vi "Test - 7.vi"() -> ()   [LabVIEW 2013]
uses:
  Item/Ctls/Item Reference.ctl
  Channel/Ctls/ChannelSetting.ctl
  Channel/Ctls/IOType.ctl
  Channel/Ctls/Dimensions.ctl
  <vilib>/Utility/sysdir.llb/System Directory Type.ctl
  Section/Section.lvclass
  Channel/Channel.lvclass
  Item/Item.lvclass
panel:
  in  "树形":string(tree)
  out "Property Names":string[](array[string])
  out "Values":variant[](array[variant])
  out "Children Item Names":string[](array[string])
  out "Newly Created?":bool
  in  "刷新按钮":bool
  in  "Name":string
  out "found":bool
  out "PathName":string
  out "Address":string
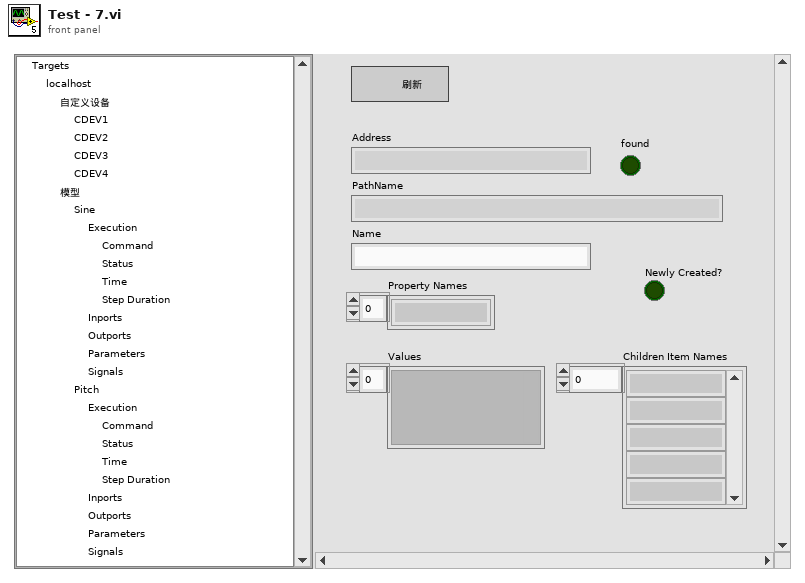
[diagram p1: front panel]
types:
  T1 = typedef "Hierarchy Framework.lvlib/Item.lvclass/Item Reference.ctl" = u64
  T2 = cluster{"Left Cell String":string, "Child Text":string[], "Child Tag":string, "Item Indent":i32, "Child Only?":bool, "Glyph Index":i32}[]
  T3 = cluster{"SectionName":string, "TypeGUID":string}[]
  T4 = typedef "Hierarchy Framework.lvlib/Channel.lvclass/ChannelSetting.ctl" = cluster{"IOType":T5, "DefaultValue":dbl[][], "Dimensions":T6, "Units":string, "Description":string, "Faultable":bool}
  T5 = typedef "Hierarchy Framework.lvlib/Channel.lvclass/IOType.ctl" = enum16{"Input", "Output"}
  T6 = typedef "Hierarchy Framework.lvlib/Channel.lvclass/Dimensions.ctl" = cluster{"Row":i32, "Column":i32}
  T7 = cluster{"Channel Name":string, "Channel Setting":T4}[]
  T8 = typedef "System Directory Type.ctl" = i32
  T9 = typedef "Hierarchy Framework.lvlib/Item.lvclass/Item Info.ctl" = cluster{"Name":string, "TagGUID":string, "TypeGUID":string, "Enable":bool}
  T10 = typedef "LVPoint32TypeDef.ctl" = cluster{"Horizontal":i32, "Vertical":i32}
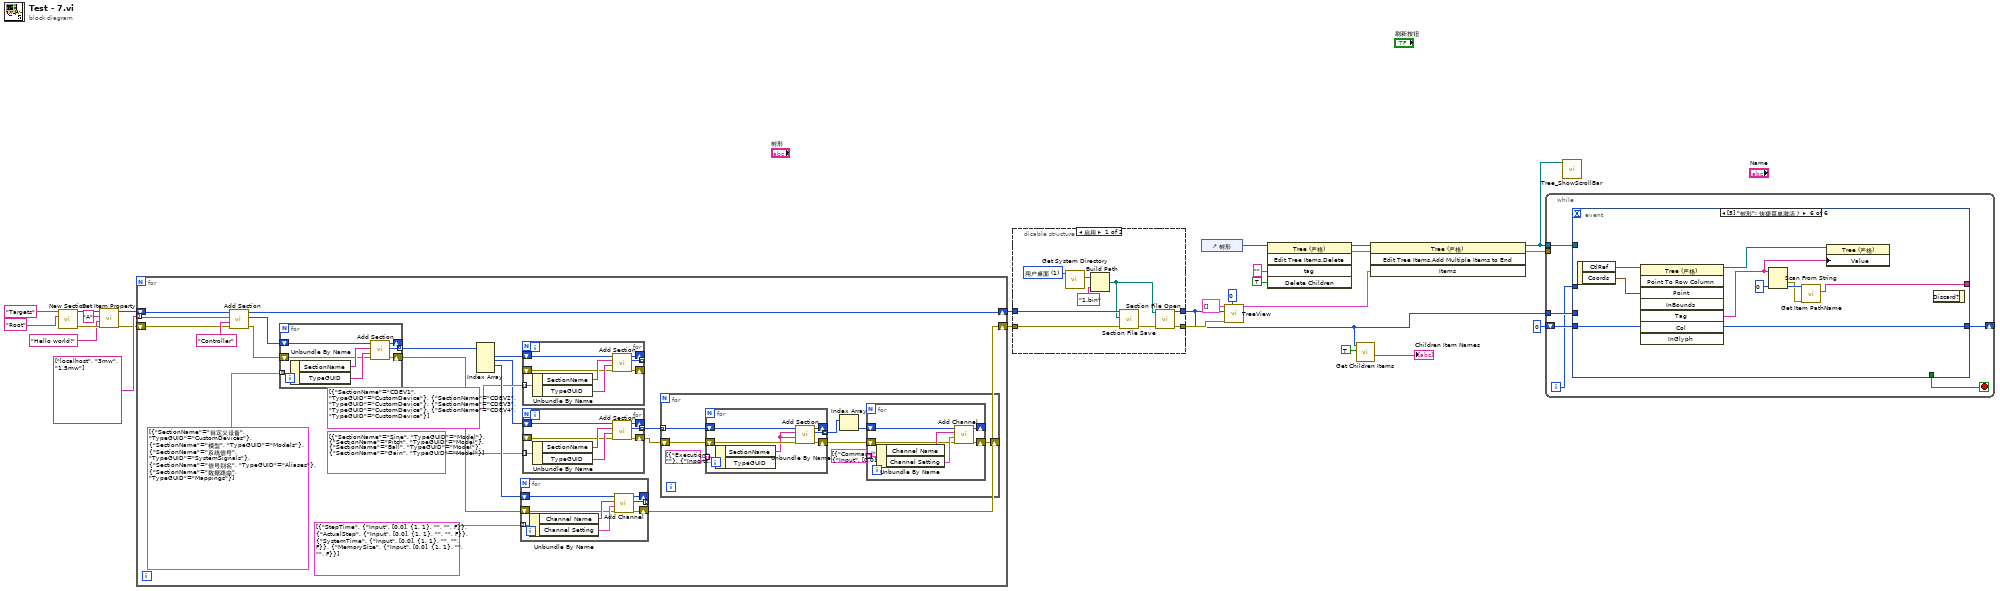
[diagram p0: block diagram]
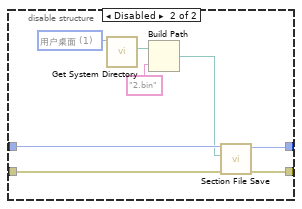
[diagram p2: hidden frame]
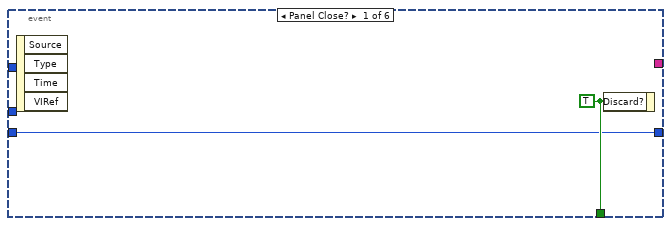
[diagram p3: hidden frame]
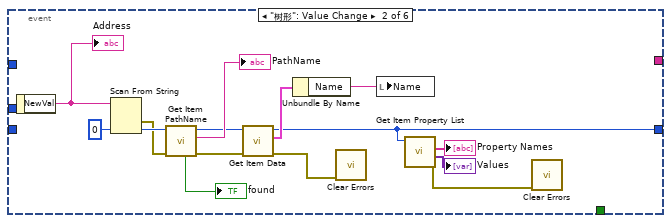
[diagram p4: hidden frame]
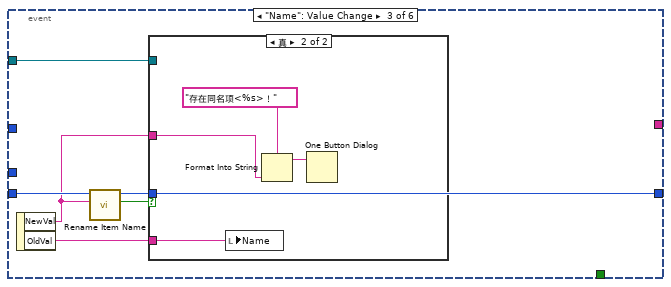
[diagram p5: hidden frame]
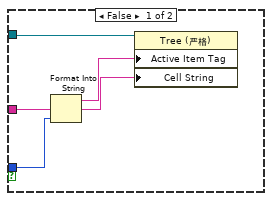
[diagram p6: hidden frame]
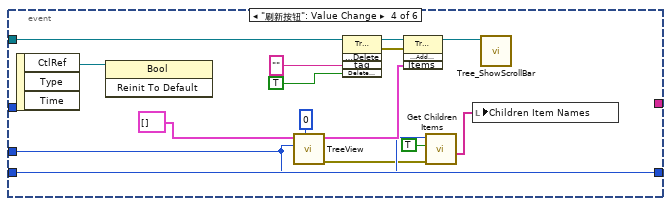
[diagram p7: hidden frame]
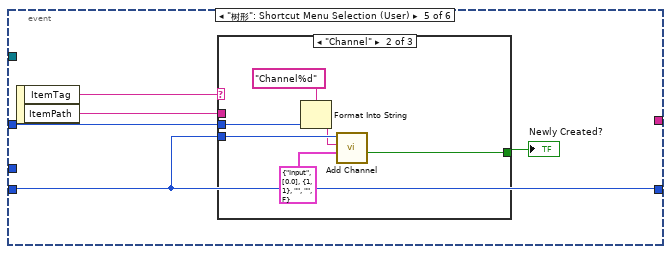
[diagram p8: hidden frame]
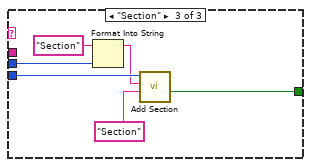
[diagram p10: hidden frame]
diagram:
  n1 = call "New Section.vi"("TypeGUID"="Root" ("Name"), "Name"="Targets") -> ("error out"=w6:errorcluster, "Section Reference in"=w8:u64)  [unwired: 8 in]
  n2 = call "Set Item Property.vi"("error in (no error)"=w6, "Value"="Hello world!" ("Property Name"), "Property Name"="A", "Item Reference in"=w8) -> ("error out"=w5:errorcluster, "Item Reference out"=w7:T1)  [unwired: 5 in, 1 out]
  n3 = for {
    shift-right: [w37] -> w2
    shift-left: w7 -> [w35]
    shift-right: [w36] -> w10
    shift-left: w5 -> [w34]
    tunnel: string[] ["localhost", "3mw", "1.5mw"] -> [w33] mode=indexing
    n4 = call "Add Section.vi"("error in (no error)"=w34, "TypeGUID"="Controller" ("SectionName"), "SectionName"=w33, "Section Reference in"=w35) -> ("error out"=w39:errorcluster, "Section Reference"=w44:u64, "Section Reference out"=w37:u64)  [unwired: 4 in, 1 out]
    n5 = for {
      shift-right: [w98] -> _
      shift-left: w44 -> [w99]
      tunnel: T3 [{"SectionName"="自定义设备", "TypeGUID"="CustomDevices"}, {"SectionName"="模型", "TypeGUID"="Models"}, {"SectionName"="系统信号", "TypeGUID"="SystemSignals"}, {"SectionName"="信号别名", "TypeGUID"="Aliases"}, {"SectionName"="数据路由", "TypeGUID"="Mappings"}] -> [w97] mode=indexing
      tunnel: [w94] -> w42 mode=indexing
      shift-right: [w92] -> w38
      shift-left: w39 -> [w93]
      n6 = Unbundle By Name(w97) -> ("SectionName"=w96:string, "TypeGUID"=w95:string)
      n7 = call "Add Section.vi"("error in (no error)"=w93, "TypeGUID"=w95, "SectionName"=w96, "Section Reference in"=w99) -> ("error out"=w92:errorcluster, "Section Reference"=w94:u64, "Section Reference out"=w98:u64)  [unwired: 4 in, 1 out]
    }
    n8 = Index Array(array=w42) -> (element #1=w32:u64, element #2=w30:u64, element #3=w40:u64)  [unwired: 4 in, 1 out]
    n9 = for {
      shift-right: [w90] -> _
      shift-left: w40 -> [w91]
      tunnel: T7 [{"Channel Name"="StepTime", "Channel Setting"={"IOType"=enum."Input", "DefaultValue"=[[0.0]], "Dimensions"={"Row"=1, "Column"=1}, "Units"="", "Description"="", "Faultable"=FALSE}}, {"Channel Name"="ActualStep", "Channel Setting"={"IOType"=enum."Input", "DefaultValue"=[[0.0]], "Dimensions"={"Row"=1, "Column"=1}, "Units"="", "Description"="", "Faultable"=FALSE}}, {"Channel Name"="SystemTime", "Channel Setting"={"IOType"=enum."Input", "DefaultValue"=[[0.0]], "Dimensions"={"Row"=1, "Column"=1}, "Units"="", "Description"="", "Faultable"=FALSE}}, {"Channel Name"="MemorySize", "Channel Setting"={"IOType"=enum."Input", "DefaultValue"=[[0.0]], "Dimensions"={"Row"=1, "Column"=1}, "Units"="", "Description"="", "Faultable"=FALSE}}] -> [w89] mode=indexing
      tunnel: [w86] -> _ mode=indexing
      shift-right: [w84] -> w36
      shift-left: w38 -> [w85]
      n10 = Unbundle By Name(w89) -> ("Channel Name"=w88:string, "Channel Setting"=w87:T4)
      n11 = call "Add Channel.vi"("error in (no error)"=w85, "Channel Setting"=w87, "Channel Name"=w88, "Section Reference in"=w91) -> ("error out"=w84:errorcluster, "Channel Reference"=w86:u64, "Section Reference out"=w90:u64)  [unwired: 4 in, 1 out]
    }
    n12 = for {
      shift-right: [w82] -> _
      shift-left: w32 -> [w83]
      tunnel: T3 [{"SectionName"="CDEV1", "TypeGUID"="CustomDevice"}, {"SectionName"="CDEV2", "TypeGUID"="CustomDevice"}, {"SectionName"="CDEV3", "TypeGUID"="CustomDevice"}, {"SectionName"="CDEV4", "TypeGUID"="CustomDevice"}] -> [w81] mode=indexing
      tunnel: [w78] -> _ mode=indexing
      shift-right: [w76] -> _
      shift-left: _ -> [w77]
      n13 = Unbundle By Name(w81) -> ("SectionName"=w80:string, "TypeGUID"=w79:string)
      n14 = call "Add Section.vi"("error in (no error)"=w77, "TypeGUID"=w79, "SectionName"=w80, "Section Reference in"=w83) -> ("error out"=w76:errorcluster, "Section Reference"=w78:u64, "Section Reference out"=w82:u64)  [unwired: 4 in, 1 out]
    }
    n15 = for {
      shift-right: [w74] -> _
      shift-left: w30 -> [w75]
      tunnel: T3 [{"SectionName"="Sine", "TypeGUID"="Model"}, {"SectionName"="Pitch", "TypeGUID"="Model"}, {"SectionName"="Ball", "TypeGUID"="Model"}, {"SectionName"="Gain", "TypeGUID"="Model"}] -> [w73] mode=indexing
      tunnel: [w70] -> w28 mode=indexing
      shift-right: [w68] -> w27
      shift-left: _ -> [w69]
      n16 = Unbundle By Name(w73) -> ("SectionName"=w72:string, "TypeGUID"=w71:string)
      n17 = call "Add Section.vi"("error in (no error)"=w69, "TypeGUID"=w71, "SectionName"=w72, "Section Reference in"=w75) -> ("error out"=w68:errorcluster, "Section Reference"=w70:u64, "Section Reference out"=w74:u64)  [unwired: 4 in, 1 out]
    }
    n18 = for {
      tunnel: w28 -> [w53] mode=indexing
      shift-right: [w46] -> _
      shift-left: w27 -> [w52]
      n19 = for {
        shift-right: [w66] -> _
        shift-left: w53 -> [w67]
        tunnel: T3 [{"SectionName"="Execution", "TypeGUID"=""}, {"SectionName"="Inports", "TypeGUID"=""}, {"SectionName"="Outports", "TypeGUID"=""}, {"SectionName"="Parameters", "TypeGUID"=""}, {"SectionName"="Signals", "TypeGUID"=""}] -> [w65] mode=indexing
        tunnel: [w64] -> w50 mode=indexing
        shift-right: [w62] -> w47
        shift-left: w52 -> [w63]
        n20 = Unbundle By Name(w65) -> ("SectionName"=w61:string)  [unwired: 1 out]
        n21 = call "Add Section.vi"("error in (no error)"=w63, "TypeGUID"=w61, "SectionName"=w61, "Section Reference in"=w67) -> ("error out"=w62:errorcluster, "Section Reference"=w64:u64, "Section Reference out"=w66:u64)  [unwired: 4 in, 1 out]
      }
      n22 = Index Array(array=w50) -> (element=w49:u64)  [unwired: 1 in]
      n23 = for {
        shift-right: [w59] -> _
        shift-left: w49 -> [w60]
        tunnel: T7 [{"Channel Name"="Command", "Channel Setting"={"IOType"=enum."Input", "DefaultValue"=[[0.0]], "Dimensions"={"Row"=1, "Column"=1}, "Units"="", "Description"="", "Faultable"=FALSE}}, {"Channel Name"="Status", "Channel Setting"={"IOType"=enum."Input", "DefaultValue"=[[0.0]], "Dimensions"={"Row"=1, "Column"=1}, "Units"="", "Description"="", "Faultable"=FALSE}}, {"Channel Name"="Time", "Channel Setting"={"IOType"=enum."Input", "DefaultValue"=[[0.0]], "Dimensions"={"Row"=1, "Column"=1}, "Units"="", "Description"="", "Faultable"=FALSE}}, {"Channel Name"="Step Duration", "Channel Setting"={"IOType"=enum."Input", "DefaultValue"=[[0.0]], "Dimensions"={"Row"=1, "Column"=1}, "Units"="", "Description"="", "Faultable"=FALSE}}] -> [w58] mode=indexing
        shift-right: [w54] -> w46
        shift-left: w47 -> [w55]
        n24 = Unbundle By Name(w58) -> ("Channel Name"=w57:string, "Channel Setting"=w56:T4)
        n25 = call "Add Channel.vi"("error in (no error)"=w55, "Channel Setting"=w56, "Channel Name"=w57, "Section Reference in"=w60) -> ("error out"=w54:errorcluster, "Section Reference out"=w59:u64)  [unwired: 4 in, 2 out]
      }
    }
  }
  n26 = disable-structure shown="启用" {
    disable-tunnel: [w108 w112] -> w1
    disable-tunnel: w2 -> [w104 w113]
    disable-tunnel: w10 -> [w103 w111]
    disable-tunnel: [w100 w110] -> w9
    frame Enabled {
      w105 = T8 1 items=["用户目录"=0, "用户桌面"=1, "用户文档"=2, "用户应用程序数据"=3, "用户设置"=4, "用户临时目录"=5, "公共文档"=6, "公共应用程序数据"=7, "公共设置"=8, "公共缓存"=13, "系统核心库"=9, "系统安装库"=10, "应用程序文件"=11, "启动盘根目录"=12] ("system directory type")
      n27 = call <vilib>:"Get System Directory.vi"("system directory type"=w105) -> ("system directory"=w106:path)  [unwired: 10 in]
      n28 = Build Path(base path=w106, name or relative path="1.bin" ("名称或相对路径")) -> (appended path=w101:path)
      n29 = call "Section File Save.vi"("error in (no error)"=w103, "Section File Path"=w101, "Section Reference in"=w104) -> ("error out"=w102:errorcluster)  [unwired: 7 in, 1 out]
      n30 = call "Section File Open.vi"("error in (no error)"=w102, "Section File Path"=w101) -> ("error out"=w100:errorcluster, "Section Reference out"=w108:u64)  [unwired: 8 in]
    }
    frame Disabled {
      w114 = T8 1 items=["用户目录"=0, "用户桌面"=1, "用户文档"=2, "用户应用程序数据"=3, "用户设置"=4, "用户临时目录"=5, "公共文档"=6, "公共应用程序数据"=7, "公共设置"=8, "公共缓存"=13, "系统核心库"=9, "系统安装库"=10, "应用程序文件"=11, "启动盘根目录"=12] ("system directory type")
      n31 = call <vilib>:"Get System Directory.vi"("system directory type"=w114) -> ("system directory"=w115:path)  [unwired: 10 in]
      n32 = Build Path(base path=w115, name or relative path="2.bin" ("名称或相对路径")) -> (appended path=w109:path)
      n33 = call "Section File Save.vi"("error in (no error)"=w111, "Section File Path"=w109, "Section Reference in"=w113) -> ("error out"=w110:errorcluster, "Section Reference out"=w112:u64)  [unwired: 7 in]
    }
  }
  n34 = control-ref of="树形"() -> (w26:refnum<vi>)
  n35 = call "TreeView.vi"("Item Indent"=0, "error in (no error)"=w9, "Item Reference in"=w1, "Items in"=T2 []) -> ("Items out"=w19:T2)  [unwired: 6 in, 1 out]
  n36 = invoke class="Tree (严格)" method="Edit Tree Items.Delete"(reference=w26, "tag"="" ("标识符"), "Delete Children"=TRUE ("删除子项？")) -> (reference out=w20:refnum<vi>, error out=w21:errorcluster)  [unwired: 2 in, 3 out]
  n37 = call "Get Children Items.vi"("Whole Hierarchy?(F)"=TRUE ("Whole Indent?(F)"), "Section Reference in"=w1) -> ("Children Item Names"=→"Children Item Names":string[])  [unwired: 5 in, 4 out]
  n38 = invoke class="Tree (严格)" method="Edit Tree Items.Add Multiple Items to End"(reference=w20, error in=w21, "Items"=w19) -> (reference out=w13:refnum<vi>, error out=w17:errorcluster)  [unwired: 1 in, 2 out]
  n39 = while {
    tunnel: w17 -> [_]
    shift-right: [w121] -> _
    shift-left: T1 0 ("Item Reference out") -> [w120]
    tunnel: w13 -> [w119]
    tunnel: w1 -> [w118]
    i -> [w117]
    stop <- w122 stop-if-true
    n40 = event shown="[5] \"树形\": 快捷菜单激活？" {
      selector: _ -> [_ _ _ _ _ _]
      dyn-events: _ -> [_ _ _ _ _ _]
      timeout: _ -> [_ _ _ _ _ _]
      tunnel: [w124 _ _ _ _ _] -> w122
      tunnel: [w123 w126 w142 w168 w172 w194] -> w121
      tunnel: w120 -> [w123 _ w145 w168 w172 w194]
      tunnel: w119 -> [_ _ w143 w160 _ _]
      tunnel: w118 -> [_ _ _ w156 _ _]
      tunnel: w117 -> [_ _ _ _ w171 _]
      tunnel: [_ _ _ _ _ w187] -> _
      event Panel Close? {
        w124 = TRUE ("放弃？")
        n41 = event-data() -> ()  [unwired: 1 in, 4 out]
        n42 = event-data("Discard?"=w124) -> ()  [unwired: 1 in, 1 out]
      }
      event "树形": Value Change {
        n43 = event-data() -> ("NewVal"=w139:string)  [unwired: 1 in]
        "Address" <- w139
        n44 = Scan From String(input string=w139, default 1=u64 0 ("默认值 1")) -> (error out=w134:errorcluster, output 1=w137:u64)  [unwired: 3 in, 2 out]
        n45 = call "Get Item PathName.vi"("error in (no error)"=w134, "Item Reference in"=w137) -> ("error out"=w132:errorcluster, "PathName"=→"PathName":string, "Item Reference out"=w133:T1, "found"=→"found":bool)  [unwired: 6 in]
        n46 = call "Get Item Data.vi"("error in (no error)"=w132, "Item Reference in"=w133) -> ("error out"=w131:errorcluster, "Item Info"=w130:T9, "Item Reference out"=w126:T1)  [unwired: 6 in, 1 out]
        n47 = Unbundle By Name(w130) -> ("Name"=w129:string)
        n48 = call <vilib>:"Clear Errors.vi"("error in (no error)"=w131) -> ()  [unwired: 6 in, 1 out]
        n49 = local write "Name"(w129) -> ()
        n50 = call "Get Item Property List.vi"("Item Reference in"=w126) -> ("error out"=w125:errorcluster, "Values"=→"Values":variant[], "Property Names"=→"Property Names":string[])  [unwired: 7 in, 1 out]
        n51 = call <vilib>:"Clear Errors.vi"("error in (no error)"=w125) -> ()  [unwired: 6 in, 1 out]
      }
      event "Name": Value Change {
        n52 = event-data() -> ("NewVal"=w141:string, "OldVal"=w140:string)  [unwired: 1 in]
        n53 = call "Rename Item Name.vi"("New Name"=w141, "Item Reference in"=w145) -> ("Request invalid?"=w144:bool, "Item Reference out"=w142:T1)  [unwired: 7 in, 1 out]
        n54 = case shown="真" w144 {
          tunnel: w143 -> [w149 _]
          tunnel: w142 -> [w148 _]
          tunnel: w141 -> [w146 w150]
          tunnel: w140 -> [_ w152]
          frame False {
            n55 = Format Into String(w148) -> (resulting string=w147:string)  [unwired: 3 in, 1 out]
            n56 = property class="Tree (严格)"(reference=w149, "Active Item Tag"=w147, "Cell String"=w146) -> ()  [unwired: 1 in, 2 out]
          }
          frame True {
            n57 = local write "Name"(w152) -> ()
            n58 = Format Into String(format string="存在同名项<%s>！" ("消息"), w150) -> (resulting string=w151:string)  [unwired: 2 in, 1 out]
            n59 = One Button Dialog(message=w151) -> ()  [unwired: 1 in, 1 out]
          }
        }
      }
      event "刷新按钮": Value Change {
        n60 = event-data() -> ("CtlRef"=w167:refnum<vi>)  [unwired: 1 in, 2 out]
        n61 = invoke class="Bool" method="Reinit To Default"(reference=w167) -> ()  [unwired: 2 in, 3 out]
        n62 = call "TreeView.vi"("Item Indent"=0, "Item Reference in"=w156, "Items in"=T2 []) -> ("error out"=w155:errorcluster, "Items out"=w159:T2)  [unwired: 7 in]
        n63 = invoke class="Tree (严格)" method="Edit Tree Items.Delete"(reference=w160, "tag"="" ("标识符"), "Delete Children"=TRUE ("删除子项？")) -> (reference out=w161:refnum<vi>, error out=w162:errorcluster)  [unwired: 2 in, 3 out]
        n64 = invoke class="Tree (严格)" method="Edit Tree Items.Add Multiple Items to End"(reference=w161, error in=w162, "Items"=w159) -> (reference out=w158:refnum<vi>)  [unwired: 1 in, 3 out]
        n65 = call "Get Children Items.vi"("error in (no error)"=w155, "Whole Hierarchy?(F)"=TRUE ("Whole Indent?(F)"), "Section Reference in"=w156) -> ("Children Item Names"=w154:string[])  [unwired: 4 in, 4 out]
        n66 = local write "Children Item Names"(w154) -> ()
        n67 = call <vilib>:"Tree_ShowScrollBar.vi"("Tree"=w158) -> ()  [unwired: 10 in, 1 out]
      }
      event "树形": Shortcut Menu Selection (User) {
        n68 = event-data() -> ("ItemTag"=w173:string, "ItemPath"=w170:string)  [unwired: 1 in]
        n69 = case shown="\"Channel\"" w173 {
          tunnel: w172 -> [_ w179 w185]
          tunnel: w171 -> [_ w175 w182]
          tunnel: [_ w174 w180] -> w169
          tunnel: w170 -> [_ _ _]
          frame "假", Default {
          }
          frame "Channel" {
            n70 = Format Into String(format string="Channel%d" ("Channel Name"), w175) -> (resulting string=w176:string)  [unwired: 2 in, 1 out]
            n71 = call "Add Channel.vi"("Channel Setting"=T4 {"IOType"=enum."Input", "DefaultValue"=[[0.0]], "Dimensions"={"Row"=1, "Column"=1}, "Units"="", "Description"="", "Faultable"=FALSE}, "Channel Name"=w176, "Section Reference in"=w179) -> ("Newly Created?"=w174:bool)  [unwired: 5 in, 3 out]
          }
          frame "Section" {
            n72 = Format Into String(initial string="Section" ("初始字符串"), w182) -> (resulting string=w183:string)  [unwired: 2 in, 1 out]
            n73 = call "Add Section.vi"("TypeGUID"="Section", "SectionName"=w183, "Section Reference in"=w185) -> ("Newly Created?"=w180:bool)  [unwired: 5 in, 3 out]
          }
        }
        "Newly Created?" <- w169
      }
      event "树形": Shortcut Menu Activation? {
        n74 = event-data() -> ("CtlRef"=w193:refnum<vi>, "Coords"=w192:T10)  [unwired: 1 in]
        n75 = invoke class="Tree (严格)" method="Point To Row Column"(reference=w193, "Point"=w192) -> (reference out=w188:refnum<vi>, "Tag"=w186:string)  [unwired: 6 in, 6 out]
        n76 = Scan From String(input string=w186, default 1=u64 0 ("默认值 1")) -> (error out=w189:errorcluster, output 1=w190:u64)  [unwired: 3 in, 2 out]
        n77 = call "Get Item PathName.vi"("error in (no error)"=w189, "Item Reference in"=w190) -> ("PathName"=w187:string)  [unwired: 6 in, 3 out]
        n78 = property class="Tree (严格)"(reference=w188, "Value"=w186) -> ()  [unwired: 1 in, 2 out]
        n79 = event-data() -> ()  [unwired: 2 in, 1 out]
      }
    }
  }
  n80 = call <vilib>:"Tree_ShowScrollBar.vi"("Tree"=w13) -> ()  [unwired: 10 in, 1 out]
